vi "Open Device.vi"(8 "error in (no error)":errorcluster, 11 "Simulated Waveform in":refnum<class "Simulated Waveform.lvclass">) -> (0 "error out":errorcluster, 3 "Simulated Waveform out":refnum<class "Simulated Waveform.lvclass">)   [LabVIEW 2020, in "Simulated Waveform.lvlib" / "Simulated Waveform.lvclass"]
uses:
  Simulated Waveform.lvclass
  Simulated Waveform.lvclass/Simulated Waveform.ctl
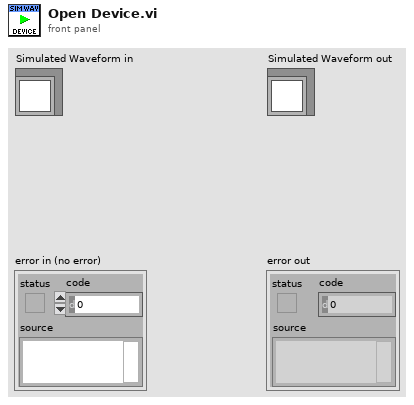
[diagram p1: front panel]
types:
  T1 = typedef "Simulated Waveform.lvlib/Simulated Waveform.lvclass/Ref Data.ctl" = cluster{"Sim Queue Name":string, "Waveform Queue":refnum<queue>, "Noise Factor":dbl}
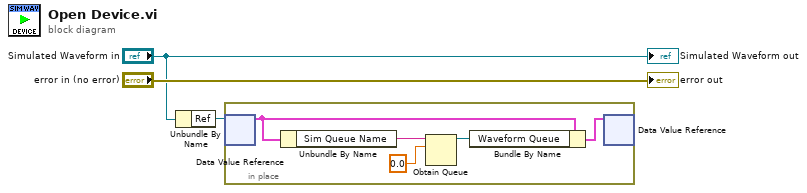
[diagram p0: block diagram]
diagram:
  n1 = Unbundle By Name("Simulated Waveform in") -> ("Ref"=w2:refnum<data-value>)
  n2 = in-place {
    n3 = in-place-dvr #1(w2) -> (w6:T1)  [unwired: 1 out]
    n4 = Unbundle By Name(w6) -> ("Sim Queue Name"=w7:string)
    n5 = Obtain Queue(name (unnamed)=w7, element data type=0.0) -> (queue out=w5:refnum<queue>)  [unwired: 3 in, 2 out]
    n6 = Bundle By Name(cluster=w6, "Waveform Queue"=w5) -> (w4:T1)
    n7 = in-place-dvr #1(w4) -> ()  [unwired: 2 out]
  }
  "error out" <- "error in (no error)"
  "Simulated Waveform out" <- "Simulated Waveform in"
